vi "MT Demodulate QAM.vi"(0 "input complex waveform":T3={"t0"=0.0, "dt"=1.0, "Y"=[]} {"Y" format="%.3f"; "dt" format="%^.2e"; "t0" format="%.4f"}, 5 "QAM system parameters":T2={"samples per symbol (16)"=16, "symbol map"=[]} {"symbol map" format="%.3f"}, 7 "matched filter coefficients":dbl[](array[numeric]) format="%.2f", 9 "synchronization parameters":T1 {"sync sequence" format="%.2f"}, 11 "error in (no error)":errorcluster, 13 "reset? (T)":bool=TRUE) -> (4 "recovered complex waveform":T3 {"Y" format="%.3f"; "dt" format="%^.2e"; "t0" format="%.4f"}, 6 "output bit stream":i8[](array[numeric]), 8 "measurements":T4 {"phase offset (deg)" format="%.2f"; "frequency drift (Hz)" format="%.2f"; "frequency offset (Hz)" format="%.2f"}, 10 "sync found index (symbols)":dbl format="%.4f", 15 "error out":errorcluster)   [LabVIEW 2020, in "niDMT.lvlib"]
doc: "Demodulates a quadrature-amplitude modulation (QAM)-modulated complex baseband waveform and returns the time-aligned oversampled complex waveform, the demodulated bit stream, and the results of offset and drift measurements. This VI attempts to remove carrier and phase offset by locking to the carrier signal."
uses:
  <vilib>/addons/Modulation/niDMT.lvlib
  <vilib>/addons/Modulation/Analog/controls/Complex Data Waveform.ctl
  <vilib>/addons/Modulation/Digital/Support/Common/mod_Apply Frequency Offset (Internal).vi
  <vilib>/addons/Modulation/Analog/MT Resample (Complex Cluster).vi
  <vilib>/addons/Modulation/Analog/support/Validators/mod_Fractional Resample Validate.vi
  <vilib>/addons/Modulation/Analog/support/Validators/mod_Check Flush State.vi
  <vilib>/addons/Modulation/Analog/support/mod_FractionalResampler.vi
  <vilib>/addons/Modulation/Analog/support/mod_Integer Rate Interpolation.vi
  <vilib>/addons/Modulation/Analog/support/Validators/mod_Validate Complex Waveform.vi
  <vilib>/addons/Modulation/Analog/support/mod_PerformResampling.vi
  <vilib>/addons/Modulation/Analog/support/Validators/mod_WFErrorHandler.vi
  <vilib>/addons/Modulation/Digital/Support/Common/mod_Truncate FIR Filter (complex).vi
  <vilib>/Utility/error.llb/Error Cluster From Error Code.vi
  <vilib>/addons/Modulation/Analog/support/mod_Resampling Factors.vi
  <vilib>/addons/Modulation/Analog/support/mod_ResamplingFilter.vi
  <vilib>/addons/Modulation/Analog/support/mod_Generate Integer Interpolation Filter.vi
  <vilib>/addons/Modulation/niAMT.lvlib
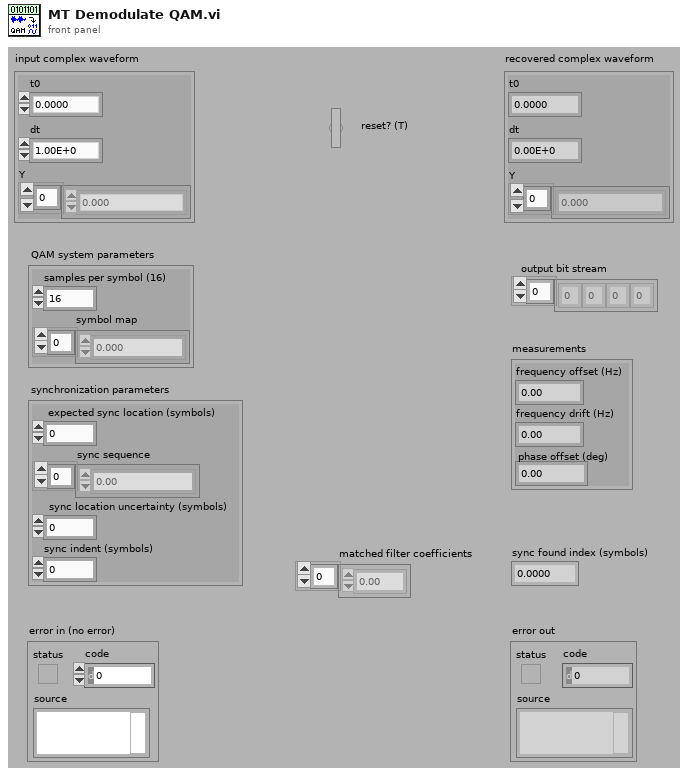
[diagram p1: front panel]
types:
  T1 = cluster{"expected sync location (symbols)":i32, "sync sequence":cdb[], "sync location uncertainty (symbols)":i32, "sync indent (symbols)":i32}
  T2 = cluster{"samples per symbol (16)":i32, "symbol map":cdb[]}
  T3 = typedef "niAMT.lvlib/Complex Data Waveform.ctl" = cluster{"t0":dbl, "dt":dbl, "Y":cdb[]}
  T4 = cluster{"frequency offset (Hz)":dbl, "frequency drift (Hz)":dbl, "phase offset (deg)":dbl}
  T5 = enum16{"FSK", "PSK", "QAM", "MSK", "PAM", "ASK", "CPM"}
  T6 = cluster{dbl, "Frequency Drift, Hz":dbl, "Phase Error Estimate, rads":dbl}
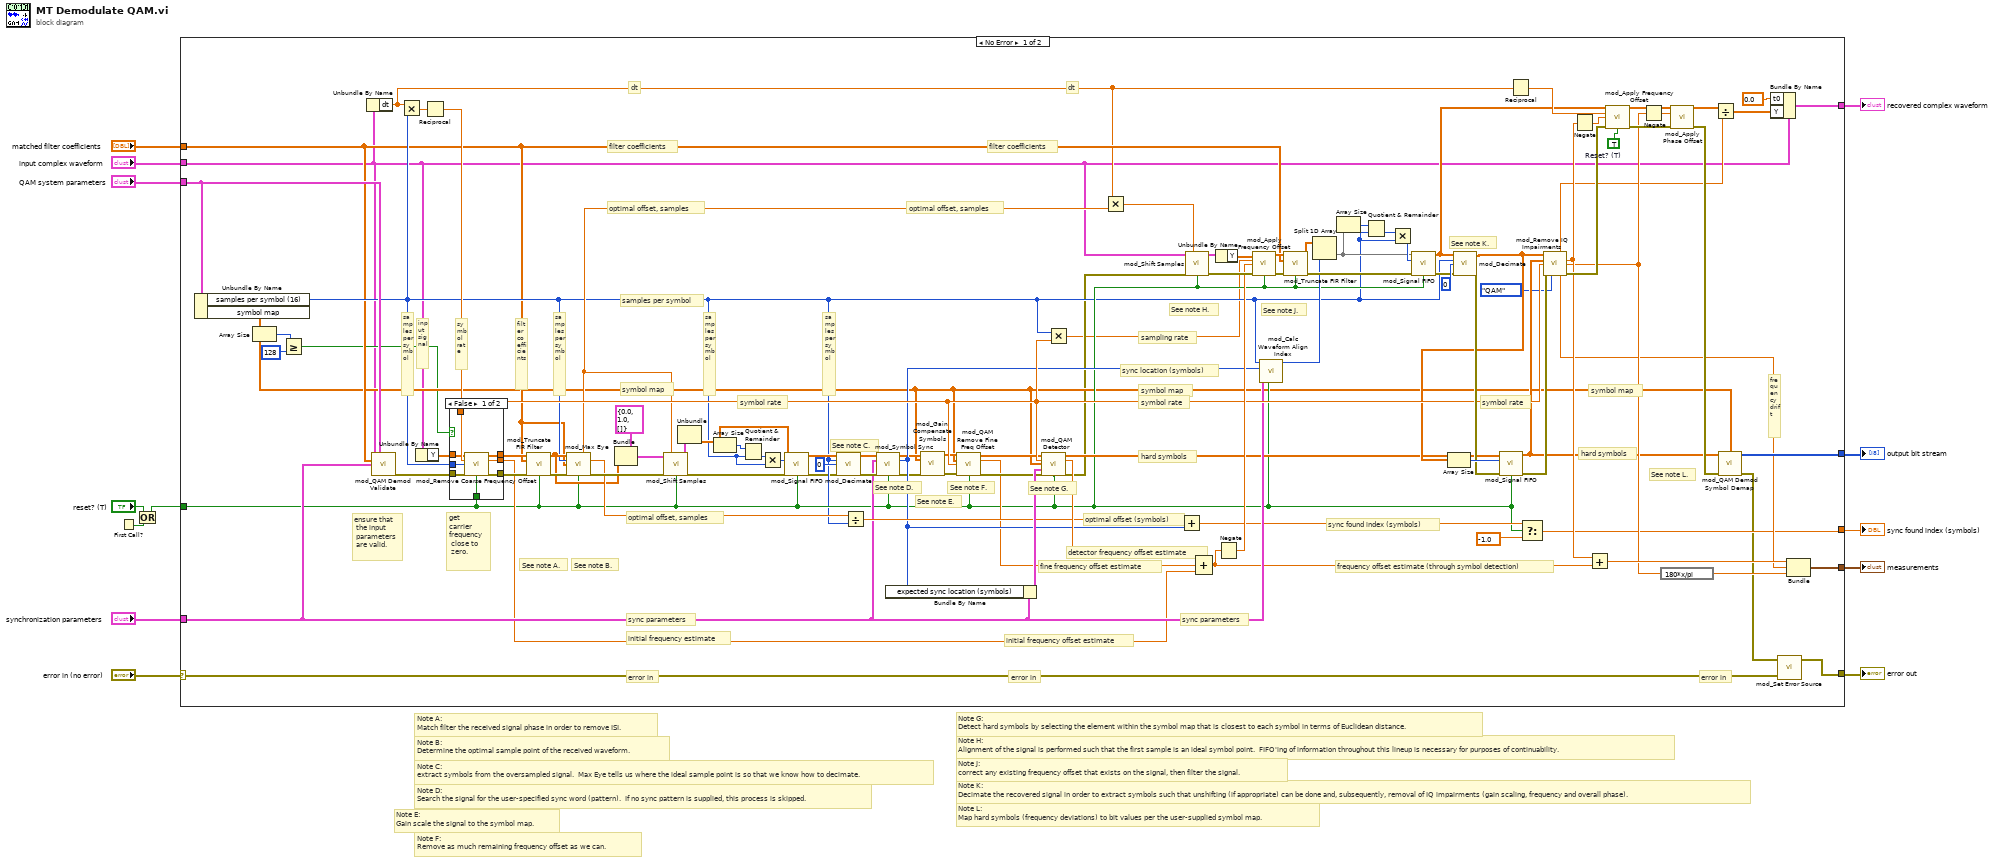
[diagram p0: block diagram]
diagram:
  # "Note E:\nGain scale the signal to the symbol map."
  # "Note L:\nMap hard symbols (frequency deviations) to bit values per the user-supplied symbol map."
  # "Note H:\nAlignment of the signal is performed such that the first sample is an ideal symbol point.  FIFO'ing of information throughout this lineup is necessary for purposes of continuability."
  # "Note D:\nSearch the signal for the user-specified sync word (pattern).  If no sync pattern is supplied, this process is skipped."
  # "Note F:\nRemove as much remaining frequency offset as we can."
  # "Note C:\nextract symbols from the oversampled signal.  Max Eye tells us where the ideal sample point is so that we know how to decimate."
  # "Note B:\nDetermine the optimal sample point of the received waveform."
  # "Note A:\nMatch filter the received signal phase in order to remove ISI."
  # "Note G:\nDetect hard symbols by selecting the element within the symbol map that is closest to each symbol in terms of Euclidean distance."
  # "Note J:\ncorrect any existing frequency offset that exists on the signal, then filter the signal."
  # "Note K:\nDecimate the recovered signal in order to extract symbols such that unshifting (if appropriate) can be done and, subsequently, removal of IQ impairments (gain scaling, frequency and overall phase)."
  n1 = First Call?() -> (First Call?: T/F=w3:bool)
  n2 = Or(x="reset? (T)", y=w3) -> (x .or. y?=w2:bool)
  n3 = case shown="No Error" "error in (no error)" {
    selector: "error in (no error)" -> [w34 w124]
    tunnel: w2 -> [w45 _]
    tunnel: "input complex waveform" -> [w16 _]
    tunnel: [w33 w124] -> w4
    tunnel: "matched filter coefficients" -> [w32 _]
    tunnel: [w113 _] -> w7
    tunnel: [w63 _] -> w6
    tunnel: [w102 _] -> w8
    tunnel: "QAM system parameters" -> [w92 _]
    tunnel: "synchronization parameters" -> [w70 _]
    tunnel: [w108 _] -> w5
    frame No Error {
      w62 = TRUE  # Reset? (T)
      # "detector frequency offset estimate"
      # "fine frequency offset estimate"
      # "See note G."
      # "frequency offset estimate (through symbol detection)"
      # "error in"
      # "frequency drift"
      # "sync found index (symbols)"
      # "hard symbols"
      # "symbol map"
      # "symbol rate"
      # "dt"
      # "dt"
      # "filter coefficients"
      # "filter coefficients"
      # "sampling rate"
      # "sync location (symbols)"
      # "symbol rate"
      # "symbol rate"
      # "hard symbols"
      # "symbol map"
      # "sync parameters"
      # "error in"
      # "initial frequency offset estimate"
      # "initial frequency estimate"
      # "sync parameters"
      # "error in"
      # "samples per symbol"
      # "samples per symbol"
      # "symbol map"
      # "samples per symbol"
      # "input signal"
      # "optimal offset, samples"
      # "samples per symbol"
      # "filter coefficients"
      # "See note E."
      # "See note L."
      # "See note K."
      # "See note J."
      # "See note H."
      # "See note D."
      # "See note F."
      # "See note C."
      # "get\ncarrier\nfrequency\n close to\n zero."
      # "ensure that\n the input\n parameters\n are valid."
      # "See note B."
      # "See note A."
      # "optimal offset (symbols)"
      # "samples per symbol"
      # "optimal offset, samples"
      # "optimal offset, samples"
      # "symbol rate"
      n4 = Unbundle By Name(w92) -> ("samples per symbol (16)"=w39:i32, "symbol map"=w21:cdb[])
      n5 = Array Size(array=w21) -> (size(s)=w18:i32)
      n6 = Greater Or Equal?(x=w18, y=128) -> (x >= y?=w19:bool)
      n7 = Unbundle By Name(w16) -> ("dt"=w17:dbl)
      n8 = call <vilib>:"mod_QAM Demod Validate.vi"("Input Complex Waveform"=w16, "QAM System Parameters"=w92, "Matched Filter Coefficients"=w32, "Synchronization Parameters"=w70) -> ("error out"=w81:errorcluster)  [unwired: 11 out]
      n9 = Multiply(x=w17, y=w39) -> (x*y=w89:dbl)
      n10 = Unbundle By Name(w16) -> ("Y"=w31:cdb[])
      n11 = Reciprocal(x=w89) -> (1/x=w72:dbl)
      n12 = case shown="False" w19 {
        tunnel: [w121 w122] -> w110
        tunnel: w81 -> [w120 w122]
        tunnel: w72 -> [w119 _]
        tunnel: [w118 _] -> w59
        tunnel: [w117 w123] -> w52
        tunnel: w45 -> [w116 _]
        tunnel: w39 -> [w115 _]
        tunnel: w31 -> [w114 w123]
        frame False {
          n13 = call <vilib>:"mod_Remove Coarse Frequency Offset.vi"("Signal In"=w114, "Symbol Rate, Hz"=w119, "Samples Per Symbol (16)"=w115, "error in (no error)"=w120, "Reset? (T)"=w116) -> ("Signal Out"=w117:cdb[], "Freq Est, Hz"=w118:dbl, "error out"=w121:errorcluster)  [unwired: 3 in, 5 out]
        }
        frame True {
        }
      }
      n14 = call-poly <vilib>:"mod_Truncate FIR Filter.vi"("Signal In"=w52, "Filter Coefficients"=w32, "error in (no error)"=w110, "Reset? (T)"=w45) -> ("Signal Out"=w50:cdb[], "error out"=w82:errorcluster)  [unwired: 8 in, 2 out]
      n15 = call <vilib>:"mod_Max Eye.vi"("Signal In"=w50, "Samples Per Symbol (16)"=w39, "Filter Coefficients"=w32, "error in (no error)"=w82, "Reset? (T)"=w45) -> ("Waveform Alignment Offset"=w53:dbl, "Optimal Offset (samples)"=w54:dbl, "error out"=w57:errorcluster)  [unwired: 8 out]
      n16 = Bundle(cluster=T3 {"t0"=0.0, "dt"=1.0, "Y"=[]} ("data waveform"), "Y"=w50) -> (w56:T3)  [unwired: 2 out]
      n17 = call <vilib>:"mod_Shift Samples.vi"("Input Complex Waveform"=w56, "Initial Sample Offset, sec"=w53, "error in (no error)"=w57, "Reset? (T)"=w45) -> ("Output Complex Waveform"=w55:T3, "error out"=w38:errorcluster)  [unwired: 10 in]
      n18 = Unbundle(w55) -> ("Y"=w40:cdb[])  [unwired: 2 out]
      n19 = Array Size(array=w40) -> (size(s)=w42:i32)
      n20 = Quotient & Remainder(x=w42, y=w39) -> (floor(x/y)=w41:i32)  [unwired: 1 out]
      n21 = Multiply(x=w41, y=w39) -> (x*y=w36:i32)
      n22 = call <vilib>:"mod_Signal FIFO.vi"("Signal In"=w40, "Output Length"=w36, "error in (no error)"=w38, "Reset? (T)"=w45) -> ("Signal Out"=w43:cdb[], "error out"=w37:errorcluster)  [unwired: 10 out]
      n23 = call <vilib>:"mod_Decimate.vi"("Signal In"=w43, "Samples Per Symbol (16)"=w39, "Offset"=0, "error in (no error)"=w37) -> ("Signal Out"=w44:cdb[], "error out"=w91:errorcluster)  [unwired: 1 in, 9 out]
      n24 = Divide(x=w54, y=w39) -> (x/y=w87:dbl)
      n25 = call <vilib>:"mod_Symbol Sync.vi"("Signal In"=w44, "Synchronization Parameters"=w70, "error in (no error)"=w91, "Reset? (T)"=w45) -> ("Signal Out"=w28:cdb[], "Sync Location (symbols)"=w69:i32, "error out"=w30:errorcluster)  [unwired: 1 in, 8 out]
      n26 = Bundle By Name(cluster=w70, "expected sync location (symbols)"=w69) -> (w104:T1)
      n27 = call <vilib>:"mod_Gain Compensate Symbols.vi"("Symbols In"=w28, "Symbol Map"=w21, "error in (no error)"=w30) -> ("Symbols Out"=w27:cdb[], "error out"=w29:errorcluster)  [unwired: 11 out]
      n28 = call <vilib>:"mod_QAM Remove Fine Freq Offset.vi"("Symbols"=w27, "Symbol Map"=w21, "Symbol Rate, Hz"=w72, "error in (no error)"=w29, "Reset? (T)"=w45) -> ("Symbols"=w61:cdb[], "Freq Est, Hz"=w60:dbl, "error out"=w66:errorcluster)  [unwired: 8 out]
      n29 = call <vilib>:"mod_QAM Detector.vi"("Signal In"=w61, "Symbol Rate, Hz"=w72, "Symbol Map"=w21, "Synchronization Parameters"=w104, "error in (no error)"=w66, "Reset? (T)"=w45) -> ("Signal Out"=w67:cdb[], "Freq Est, Hz"=w112:dbl, "error out"=w15:errorcluster)  [unwired: 2 in, 5 out]
      n30 = Multiply(x=w39, y=w72) -> (x*y=w14:dbl)
      n31 = Multiply(x=w17, y=w53) -> (x*y=w105:dbl)
      n32 = Add(x=w87, y=w69) -> (x+y=w64:dbl)
      n33 = call <vilib>:"mod_Shift Samples.vi"("Input Complex Waveform"=w16, "Initial Sample Offset, sec"=w105, "error in (no error)"=w15, "Reset? (T)"=w45) -> ("Output Complex Waveform"=w107:T3, "error out"=w106:errorcluster)  [unwired: 10 in]
      n34 = Compound Arithmetic op=ADD(w112, w60, w59) -> (w24:dbl)
      n35 = Unbundle By Name(w107) -> ("Y"=w48:cdb[])
      n36 = Negate(x=w24) -> (-x=w101:dbl)
      n37 = call <vilib>:"mod_Apply Frequency Offset.vi"("Signal In"=w48, "Rate, pts/sec"=w14, "Freq Offset, Hz"=w101, "error in (no error)"=w106, "Reset? (T)"=w45) -> ("Signal Out"=w111:cdb[], "error out"=w109:errorcluster)  [unwired: 9 out]
      n38 = call <vilib>:"mod_Calc Waveform Align Index.vi"("Reset? (T)"=w45, "Synchronization Parameters"=w70, "Sync Location, symbols"=w69, "Samples Per Symbol (16)"=w39) -> ("align index, samples"=w68:i32)  [unwired: 7 out]
      n39 = call-poly <vilib>:"mod_Truncate FIR Filter.vi"("Signal In"=w111, "Filter Coefficients"=w32, "error in (no error)"=w109, "Reset? (T)"=w45) -> ("Signal Out"=w47:cdb[], "error out"=w77:errorcluster)  [unwired: 8 in, 2 out]
      n40 = Split 1D Array(array=w47, index=w68) -> (second subarray=w51:cdb[])  [unwired: 1 out]
      n41 = Array Size(array=w51) -> (size(s)=w80:i32)
      n42 = Quotient & Remainder(x=w80, y=w39) -> (floor(x/y)=w79:i32)  [unwired: 1 out]
      n43 = Multiply(x=w79, y=w39) -> (x*y=w78:i32)
      n44 = call <vilib>:"mod_Signal FIFO.vi"("Signal In"=w51, "Output Length"=w78, "error in (no error)"=w77, "Reset? (T)"=w45) -> ("Signal Out"=w46:cdb[], "error out"=w76:errorcluster)  [unwired: 10 out]
      n45 = call <vilib>:"mod_Decimate.vi"("Signal In"=w46, "Samples Per Symbol (16)"=w39, "Offset"=0, "error in (no error)"=w76) -> ("Signal Out"=w71:cdb[], "error out"=w74:errorcluster)  [unwired: 1 in, 9 out]
      n46 = Array Size(array=w71) -> (size(s)=w75:i32)
      n47 = call <vilib>:"mod_Signal FIFO.vi"("Signal In"=w67, "Output Length"=w75, "error in (no error)"=w74, "Reset? (T)"=w45) -> ("Signal Out"=w25:cdb[], "error out"=w73:errorcluster)  [unwired: 10 out]
      n48 = Reciprocal(x=w17) -> (1/x=w88:dbl)
      n49 = Select(t=w64, s=w45, f=-1.0) -> (s? t:f=w63:dbl)
      n50 = call <vilib>:"mod_Remove IQ Impairments.vi"("Received Signal In"=w71, "Reference Signal"=w25, "Signal Rate, Hz"=w72, "error in (no error)"=w73, "Modulation Type"=T5."QAM") -> ("Gain Error Estimate"=w84:dbl, "Frequency Estimate, Hz"=w95:dbl, "Phase Error Estimate, rads"=w85:dbl, "Frequency Drift, Hz"=w83:dbl, "error out"=w98:errorcluster)  [unwired: 1 in, 5 out]
      n51 = Negate(x=w95) -> (-x=w94:dbl)
      n52 = Add(x=w95, y=w24) -> (x+y=w103:dbl)
      n53 = call <vilib>:"mod_Apply Frequency Offset.vi"("Signal In"=w46, "Rate, pts/sec"=w88, "Freq Offset, Hz"=w94, "error in (no error)"=w98, "Reset? (T)"=w62) -> ("Signal Out"=w99:cdb[], "error out"=w97:errorcluster)  [unwired: 9 out]
      n54 = Negate(x=w85) -> (-x=w90:dbl)
      n55 = expression code="180*x/pi"(w85) -> (w86:dbl)
      n56 = call <vilib>:"mod_Apply Phase Offset.vi"("Signal In"=w99, "Phase Offset, rad (0 rad)"=w90, "error in (no error)"=w97) -> ("Signal Out"=w93:cdb[], "error out"=w96:errorcluster)  [unwired: 11 out]
      n57 = Divide(x=w93, y=w84) -> (x/y=w58:cdb[])
      n58 = call <vilib>:"mod_QAM Demod Symbol Demap.vi"("Symbols In"=w25, "Symbol Map"=w21, "error in (no error)"=w96) -> ("Bits Out"=w113:i8[], "error out"=w35:errorcluster)  [unwired: 1 in, 10 out]
      n59 = Bundle By Name(cluster=w16, "t0"=0.0, "Y"=w58) -> (w102:T3)
      n60 = call <vilib>:"mod_Set Error Source.vi"("initial error in (no error)"=w34, "final error in (no error)"=w35) -> ("error out"=w33:errorcluster)  [unwired: 3 out]
      n61 = Bundle(w103, "Frequency Drift, Hz"=w83, "Phase Error Estimate, rads"=w86) -> (w108:T6)  [unwired: 1 out]
    }
    frame Error {
    }
  }
  "error out" <- w4
  "measurements" <- w5
  "sync found index (symbols)" <- w6
  "output bit stream" <- w7
  "recovered complex waveform" <- w8
